vi "U8 Reverse Bit Order.vi"(1 "U8 Data In":u8 format="%02x") -> (0 "U8 Data Out":u8 format="%02x")   [LabVIEW 2016, in "SPIVI.lvlib"]
uses:
  SPIVI.lvlib
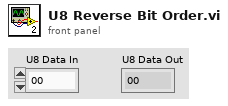
[diagram p1: front panel]
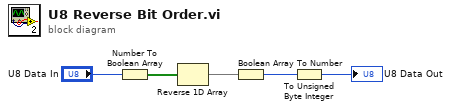
[diagram p0: block diagram]
diagram:
  n1 = Number To Boolean Array(number="U8 Data In") -> (Boolean array=w4:bool[])
  n2 = Reverse 1D Array(array=w4) -> (reversed array=w3:bool[])
  n3 = Boolean Array To Number(Boolean array=w3) -> (number=w2:u32)
  n4 = To Unsigned Byte Integer(number=w2) -> (unsigned 8bit integer=→"U8 Data Out":u8)
